vi "Load AlignmentDataCourse.vi"   [LabVIEW 2020]
uses:
  _Globals/Global Controls.vi
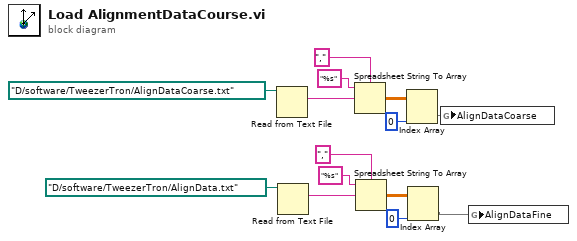
[diagram p0: block diagram]
diagram:
  n1 = Read from Text File(file (use dialog)=path "D:/software/TweezerTron/AlignDataCoarse.txt") -> (text=w13:string)  [unwired: 3 in, 3 out]
  n2 = Read from Text File(file (use dialog)=path "D:/software/TweezerTron/AlignData.txt") -> (text=w6:string)  [unwired: 3 in, 3 out]
  n3 = Spreadsheet String To Array(delimiter (Tab)=",", format string="%s", spreadsheet string=w13) -> (array=w10:dbl[][])  [unwired: 1 in]
  n4 = Spreadsheet String To Array(delimiter (Tab)=",", format string="%s", spreadsheet string=w6) -> (array=w3:dbl[][])  [unwired: 1 in]
  n5 = Index Array(array=w10, index (col)=0 ("disabled index (col)")) -> (element=w8:dbl[])  [unwired: 1 in]
  n6 = Index Array(array=w3, index (col)=0 ("disabled index (col)")) -> (element=w1:dbl[])  [unwired: 1 in]
  n7 = global write "Global Controls.vi" "AlignDataCoarse"(w8) -> ()
  n8 = global write "Global Controls.vi" "AlignDataFine"(w1) -> ()
